vi "Golden Template Inspection.vi"() -> ()   [LabVIEW 2014]
doc: "This example shows how to use the Golden Template Inspection VIs in NI Vision.\n\nThe example locates the object for inspection (a printed label) in the inspected image using Pattern Matching. Then the example compares a printed label with no defects (the golden template) with the inspected label. If the inspected label has any large defects, the label fails the inspection. The golden template file used in this example was created using the NI Vision Template Editor. The NI Vision Template Editor allows you to configure and then save information in a template file, such as the information this example used for Pattern Matching and Golden Template Inspection."
uses:
  <vilib>/vision/NI_Vision_Development_Module.lvlib
panel:
  out "Pass Status":bool
  in  "Delay (s.)":dbl(slide)=0.9924812030075187 scale=0.0..3.0
  in  "Stop":bool
  in  "Defect Display Options":T1={"Show Bright Defects"=TRUE, "Bright Color"=6618880, "Show Dark Defects"=TRUE, "Dark Color"=16711680}
  out "Inspected Image":T2(plugin-control)
  out "Golden Template":T2(plugin-control)
  # "Overview: Demonstrates how to use the IMAQ Compare Golden Template function to find areas of a printed label that don't match a golden template for the label.\nRequirements: Vision Development Software.\nInstructions: Run the VI."
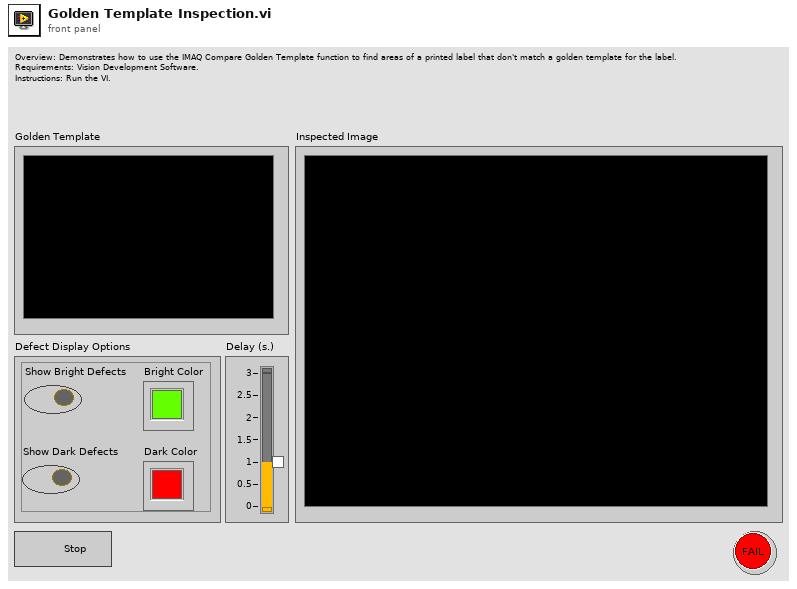
[diagram p1: front panel]
types:
  T1 = cluster{"Show Bright Defects":bool, "Bright Color":u32, "Show Dark Defects":bool, "Dark Color":u32}
  T2 = typedef "IMAQ Image.ctl" = refnum<image>
  T3 = cluster{"Position":cluster{"x":sgl, "y":sgl}, "Angle":sgl, "Scale":sgl, "Score":sgl, "Bounding Box":cluster{"x":sgl, "y":sgl}[]}[]
  T4 = cluster{"Position":cluster{"x":sgl, "y":sgl}, "Angle":sgl, "Scale":sgl, "Score":sgl, "Bounding Box":cluster{"x":sgl, "y":sgl}[]}
  T5 = cluster{"Position":cluster{"x":sgl, "y":sgl}, "Angle":sgl, "Scale":sgl}
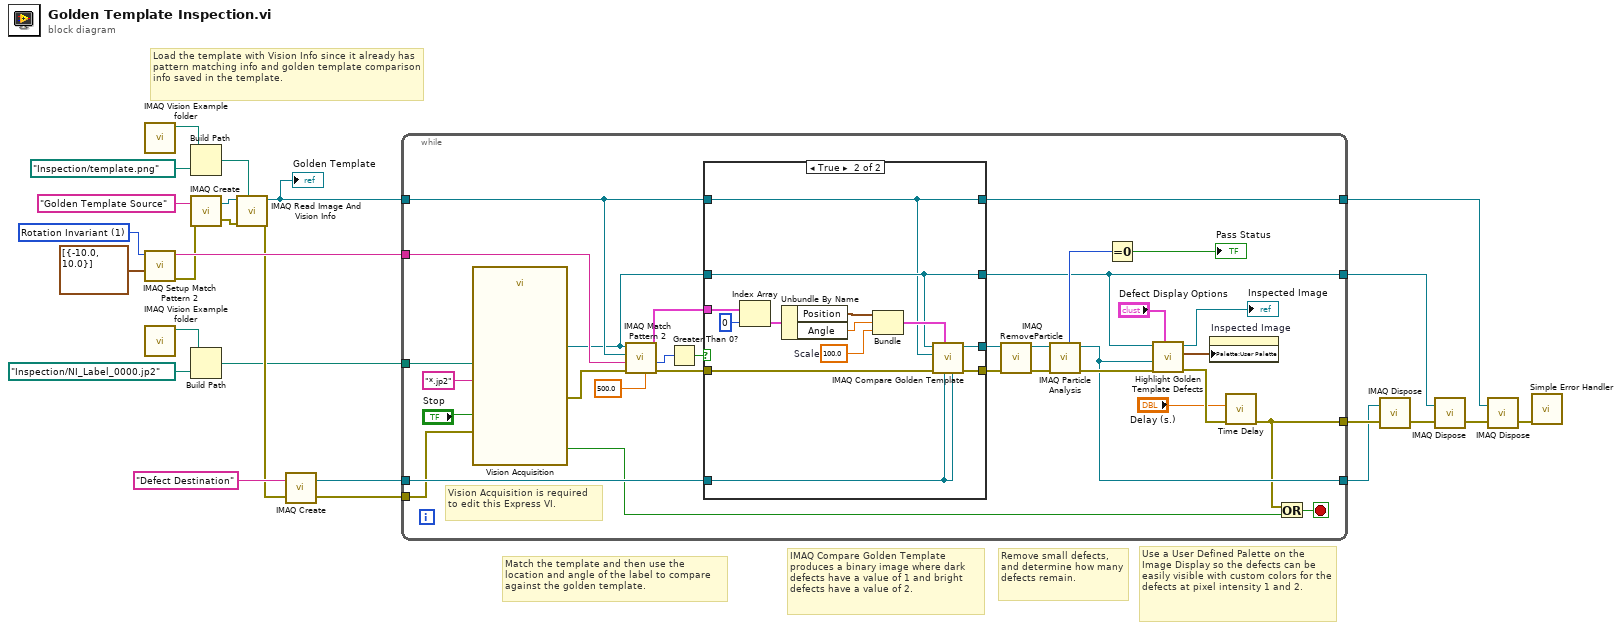
[diagram p0: block diagram]
diagram:
  w17 = u16 1 items=["Shift Invariant", "Rotation Invariant"] ("Match Mode")
  # "Use a User Defined Palette on the Image Display so the defects can be easily visible with custom colors for the defects at pixel intensity 1 and 2."
  # "Remove small defects, and determine how many defects remain."
  # "IMAQ Compare Golden Template produces a binary image where dark defects have a value of 1 and bright defects have a value of 2."
  # "Load the template with Vision Info since it already has pattern matching info and golden template comparison info saved in the template."
  # "Match the template and then use the location and angle of the label to compare against the golden template."
  n1 = call "IMAQ Vision Example folder.vi"() -> ("Example Image Path"=w18:path)  [unwired: 11 in]
  n2 = call "IMAQ Setup Match Pattern 2"("Rotation Angle Ranges (degrees)"=cluster{sgl, sgl}[] [{-10.0, 10.0}], "Match Mode"=w17) -> ("error out"=w13:errorcluster, "Match Pattern Setup Data"=w16:string)  [unwired: 3 in, 5 out]
  n3 = call "IMAQ Vision Example folder.vi"() -> ("Example Image Path"=w11:path)  [unwired: 11 in]
  n4 = Build Path(base path=w18, name or relative path=path "Inspection/template.png") -> (appended path=w22:path)
  n5 = call "IMAQ Create"("Image Name"="Golden Template Source", "error in (no error)"=w13) -> ("New Image"=w20:T2, "error out"=w14:errorcluster)  [unwired: 2 in, 1 out]
  n6 = Build Path(base path=w11, name or relative path=path "Inspection/NI_Label_0000.jp2") -> (appended path=w9:path)
  n7 = call "IMAQ Read Image And Vision Info"("File Path"=w22, "error in (no error)"=w14, "Image"=w20) -> ("error out"=w12:errorcluster, "Image Out"=w25:T2)  [unwired: 1 in, 6 out]
  "Golden Template" <- w25
  n8 = call "IMAQ Create"("Image Name"="Defect Destination", "error in (no error)"=w12) -> ("New Image"=w24:T2, "error out"=w8:errorcluster)  [unwired: 2 in, 1 out]
  n9 = while {
    tunnel: w25 -> [w57]
    tunnel: w24 -> [w56]
    tunnel: w16 -> [w55]
    tunnel: w9 -> [w47]
    tunnel: w8 -> [w46]
    tunnel: [w32] -> w2
    tunnel: [w28] -> w4
    tunnel: [w30] -> w6
    tunnel: [w29] -> w7
    stop <- w33 stop-if-true
    # "Vision Acquisition is required to edit this Express VI."
    n10 = call "Vision Acquisition"("Image Path"=w47, "Image File Type (All Types)"="*.jp2" ("pattern"), "Stop (F)"="Stop", "error in"=w46) -> ("Image Out"=w48:T2, "Stopped"=w34:bool, "error out"=w45:errorcluster)  [unwired: 21 in]
    n11 = call "IMAQ Match Pattern 2"("Minimum Match Score"=sgl 500.0, "error in (no error)"=w45, "Match Pattern Setup Data"=w55, "Template Image"=w57, "Image"=w48) -> ("error out"=w54:errorcluster, "Number of Matches"=w52:i32, "Matches"=w51:T3)  [unwired: 2 in, 2 out]
    n12 = Greater Than 0?(x=w52) -> (x > 0?=w53:bool)
    n13 = case shown="True" w53 {
      tunnel: w54 -> [w61 w62]
      tunnel: w48 -> [w60 w65]
      tunnel: w57 -> [w59 w64]
      tunnel: w51 -> [_ w73]
      tunnel: w56 -> [w58 w63]
      tunnel: [w61 w71] -> w41
      tunnel: [w58 w66] -> w31
      tunnel: [w60 w65] -> w28
      tunnel: [w59 w64] -> w32
      frame False {
      }
      frame True {
        w68 = sgl 100.0  # Scale
        n14 = Index Array(array=w73, index=0) -> (element=w72:T4)
        n15 = Unbundle By Name(w72) -> ("Position"=w70:cluster{"x":sgl, "y":sgl}, "Angle"=w69:sgl)
        n16 = Bundle("Position"=w70, "Angle"=w69, "Scale"=w68) -> (w67:T5)  [unwired: 1 in]
        n17 = call "IMAQ Compare Golden Template"("Dark Defect Image Dst"=w63, "Bright (or Both) Defect Image Dst"=w63, "Alignment"=w67, "error in (no error)"=w62, "Template Image"=w64, "Image"=w65) -> ("error out"=w71:errorcluster, "Bright (or Both) Defect Image Dst Out"=w66:T2)  [unwired: 1 in, 3 out]
      }
    }
    n18 = call "IMAQ RemoveParticle"("error in (no error)"=w41, "Image Src"=w31) -> ("error out"=w40:errorcluster, "Image Dst Out"=w43:T2)  [unwired: 5 in, 3 out]
    n19 = call "IMAQ Particle Analysis"("error in (no error)"=w40, "Image"=w43) -> ("error out"=w36:errorcluster, "Image Out (duplicate)"=w30:T2, "Number of Particles"=w42:i32)  [unwired: 3 in, 4 out]
    n20 = Equal To 0?(x=w42) -> (x = 0?=→"Pass Status":bool)
    n21 = call "Highlight Golden Template Defects.vi"("Defect Display Options"="Defect Display Options", "error in (no error)"=w36, "Defect Image"=w30, "Source Image"=w28) -> ("error out"=w35:errorcluster, "User Defined Color Palette"=w37:cluster{"Red":u8, "Green":u8, "Blue":u8}[], "Image Out"=→"Inspected Image":T2)  [unwired: 5 in]
    n22 = property on="Inspected Image" class="ImageControl"("Palette:User Palette"=w37) -> ()  [unwired: 2 in, 2 out]
    n23 = call "Time Delay"("error in (no error)"=w35, "Delay Time (s)"="Delay (s.)") -> ("error out"=w29:errorcluster)  [unwired: 9 in]
    n24 = Or(x=w29, y=w34) -> (x .or. y?=w33:bool)
  }
  n25 = call "IMAQ Dispose"("Image"=w6, "error in (no error)"=w7) -> ("error out"=w5:errorcluster)  [unwired: 4 in]
  n26 = call "IMAQ Dispose"("Image"=w4, "error in (no error)"=w5) -> ("error out"=w3:errorcluster)  [unwired: 4 in]
  n27 = call "IMAQ Dispose"("Image"=w2, "error in (no error)"=w3) -> ("error out"=w1:errorcluster)  [unwired: 4 in]
  n28 = call <vilib>:"Simple Error Handler.vi"("error in (no error)"=w1) -> ()  [unwired: 4 in, 5 out]
